vi "Keithley 3390 Frequency Sweep.vi"() -> ()   [LabVIEW 2017]
doc: "This example shows how to configure and output a frequency sweep."
uses:
  Keithley 3390.lvlib
  Public/Configure/Configure Waveform (Sine).vi
panel:
  in  "Sweep Spacing (Linear)":enum16{"Linear", "Log"}(ring)
  in  "Sweep Time (1.00 s)":dbl=1.0 format="%#.6g"
  in  "Stop  Frequency  (1000.0 Hz)":dbl=1000.0 format="%#.6g"
  in  "Start Frequency (100.0 Hz)":dbl=100.0 format="%#.6g"
  in  "Amplitude (1.0 Vpp)":dbl=1.0
  in  "VISA resource name":refnum<visa-resource-name>
  # "(c) 2008 Keithley Instruments, Inc.  ALL RIGHTS RESERVED."
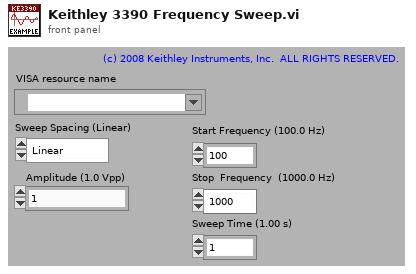
[diagram p1: front panel]
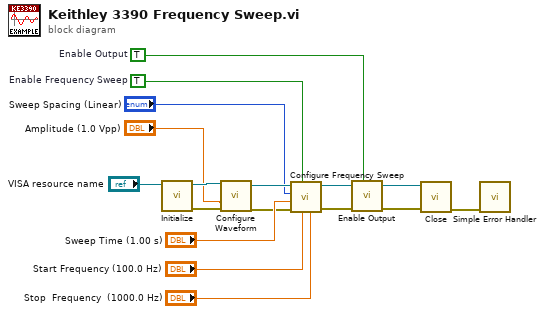
[diagram p0: block diagram]
diagram:
  w7 = TRUE  # Enable Output
  w12 = TRUE  # Enable Frequency Sweep
  n1 = call "Initialize.vi"("VISA resource name"="VISA resource name") -> ("error out"=w3:errorcluster, "VISA resource name out"=w4:refnum<visa-resource-name>)  [unwired: 9 in]
  n2 = call-poly "Configure Waveform.vi"("VISA resource name"=w4, "Amplitude (1.0 Vpp)"="Amplitude (1.0 Vpp)", "error in (no error)"=w3) -> ("VISA resource name out"=w6:refnum<visa-resource-name>, "error out"=w5:errorcluster)  [unwired: 11 in]
  n3 = call "Configure Frequency Sweep.vi"("Stop  Frequency  (1000.0 Hz)"="Stop  Frequency  (1000.0 Hz)", "Start Frequency (100.0 Hz)"="Start Frequency (100.0 Hz)", "Enable Frequency Sweep (T:Enable)"=w12, "error in (no error)"=w5, "Sweep Time (1.00 s)"="Sweep Time (1.00 s)", "Sweep Spacing (0: Linear)"="Sweep Spacing (Linear)", "VISA resource name"=w6) -> ("error out"=w10:errorcluster, "VISA resource name out"=w11:refnum<visa-resource-name>)  [unwired: 3 in]
  n4 = call "Enable Output.vi"("Enable Output (T: Enable)"=w7, "error in (no error)"=w10, "VISA resource name"=w11) -> ("error out"=w9:errorcluster, "VISA resource name out"=w8:refnum<visa-resource-name>)  [unwired: 7 in]
  n5 = call "Close.vi"("error in (no error)"=w9, "VISA resource name"=w8) -> ("error out"=w17:errorcluster)  [unwired: 9 in]
  n6 = call <vilib>:"Simple Error Handler.vi"("error in (no error)"=w17) -> ()  [unwired: 4 in, 5 out]
